vi "eec 6700 Perform Test in Manual Mode.vi"() -> ()   [LabVIEW 2014]
doc: "Configures the instrument in Manual mode and starts the test. The test meter data output is read from the instrument.\nPress stop button to end the test.\n\nNote : \n1.In firmware version 1.06, Enable Surge-Drop Mode is a system parameter (common for all steps and memory. Change in mode affect all steps and memory)\n\n2. In the firmware version 2.0 and above ,Enable Surge-Drop Mode can be used only in the Program Mode. And it can be used as a step parameter."
uses:
  <instrlib>/eec 6700/eec 6700.lvlib
panel:
  in  "Timeout (10000 ms)":u32=10000
  in  "Stop":bool
  in  "Frequency High Limit (500 Hz)":dbl=500.0 min=0.0 max=500.0 format="%.1f"
  in  "Frequency Low Limit (40 Hz)":dbl=40.0 min=0.0 max=500.0 format="%.1f"
  in  "End Angle: (0)":i32 min=0 max=359
  in  "Start Angle (0)":i32 min=0 max=359
  in  "Voltage Low Limit (0 V)":dbl min=0.0 max=400.0 format="%.1f"
  in  "Voltage High Limit (300 V)":dbl=300.0 min=0.0 max=400.0 format="%.1f"
  out "Test Meter Data Output":T1 {"Frequency (Hz)" format="%.1f"; "Voltage (V)" format="%.1f"; "RMS Current (A)" format="%.3f"; "Power (W)" format="%.1f"; "Peak Current (A)" format="%.1f"; "Power Factor" format="%.3f"; "Timer (s)" format="%.1f"}
  out "Status Byte Register Cluster":T2
  in  "Enable Surge Drop (F:Disable)":bool
  in  "Memory (1)":i32=1 min=1 max=50 step=1
  in  "Output AC Voltage Frequency (60  Hz)":dbl=60.0 min=45.0 max=500.0 format="%.1p"
  in  "Current High Limit (0 A)":dbl min=0.0 max=36.8 format="%.3f"
  in  "Output AC Voltage (115 V)":dbl=115.0 min=0.0 max=300.0 format="%.1f"
  in  "Voltage Range Mode (1:Auto)":u16(ring)=1 items=["High", "Auto"]
  in  "Surge Drop Duration (0 ms)":dbl min=0.0 max=99.0
  in  "Surge Drop Start Time (0 ms)":dbl min=0.0 max=99.0
  in  "Surge Drop Voltage (100 V)":dbl=100.0 min=0.0 max=300.0 format="%.1f"
  in  "Enable  Continuous Surge-Drop (F:Disable)":bool
  in  "Enable Over Current Fold Back (F:Disable)":bool
  in  "VISA resource name":refnum<visa-resource-name>="COM1"
  out "Error Out":errorcluster
  # "eec 6700 Manual MODE - EXAMPLE"
  # "Note :\n1. Configure the Parameters (Select the instrument VISA resource, voltage etc.,)\n2. Run this VI"
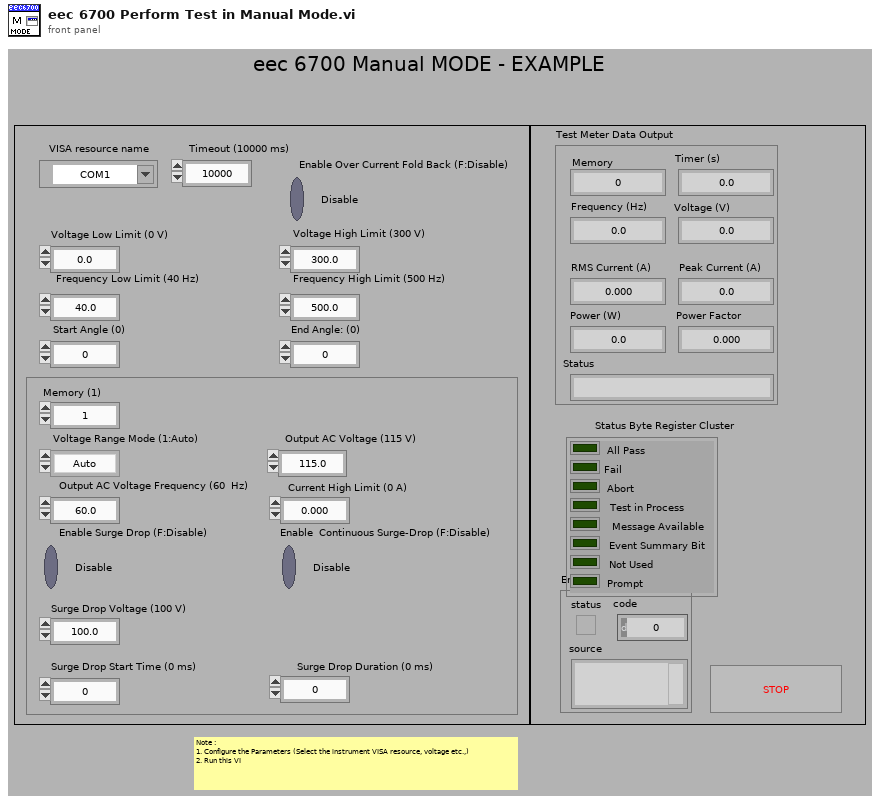
[diagram p1: front panel]
types:
  T1 = cluster{"Memory":dbl, "Timer (s)":dbl, "Frequency (Hz)":dbl, "Voltage (V)":dbl, "RMS Current (A)":dbl, "Peak Current (A)":dbl, "Power (W)":dbl, "Power Factor":dbl, "Status":string}
  T2 = cluster{"All Pass":bool, "Fail":bool, "Abort":bool, "Test in Process":bool, "Message Available":bool, "Event Summary Bit":bool, "Not Used":bool, "Prompt":bool}
  T3 = cluster{"Baud Rate":u32, "Parity":u16, "Data Bits":u16, "Stop Bits":u16, "Flow Control":u16}
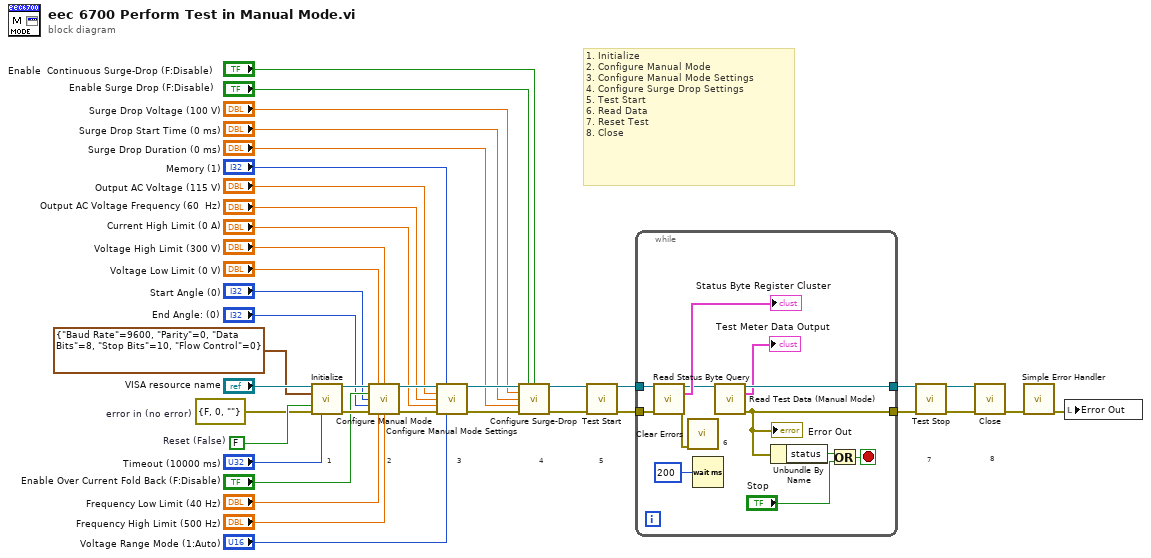
[diagram p0: block diagram]
diagram:
  w35 = errorcluster {"status"=FALSE, "code"=0, "source"=""}  # error in (no error)
  w36 = FALSE  # Reset (False)
  # "7"
  # "5"
  # "4"
  # "8"
  # "1. Initialize\n2. Configure Manual Mode\n3. Configure Manual Mode Settings\n4. Configure Surge Drop Settings\n5. Test Start\n6. Read Data\n7. Reset Test\n8. Close"
  # "3"
  # "2"
  # "1"
  n1 = call <instrlib>:"Initialize.vi"("VISA resource name"="VISA resource name", "Serial Configuration"=T3 {"Baud Rate"=9600, "Parity"=0, "Data Bits"=8, "Stop Bits"=10, "Flow Control"=0}, "Reset (True)"=w36, "error in (no error)"=w35, "Timeout (10000 ms)"="Timeout (10000 ms)") -> ("VISA resource name out"=w31:refnum<visa-resource-name>, "error out"=w33:errorcluster)  [unwired: 9 in]
  n2 = call <instrlib>:"Configure Manual Mode.vi"("VISA resource name"=w31, "Voltage Low Limit (0 V)"="Voltage Low Limit (0 V)", "Voltage High Limit (300 V)"="Voltage High Limit (300 V)", "Enable Over Current Fold Back (F:Disable)"="Enable Over Current Fold Back (F:Disable)", "Start Angle (0)"="Start Angle (0)", "End Angle: (0)"="End Angle: (0)", "error in (no error)"=w33, "Frequency Low Limit (40 Hz)"="Frequency Low Limit (40 Hz)", "Frequency High Limit (500 Hz)"="Frequency High Limit (500 Hz)") -> ("VISA resource name out"=w32:refnum<visa-resource-name>, "error out"=w34:errorcluster)  [unwired: 5 in]
  n3 = call <instrlib>:"Configure Manual Mode Settings.vi"("VISA resource name"=w32, "Memory (1)"="Memory (1)", "Output AC Voltage (115 V)"="Output AC Voltage (115 V)", "Output AC Voltage Frequency (60  Hz)"="Output AC Voltage Frequency (60  Hz)", "Current High Limit (0 A)"="Current High Limit (0 A)", "error in (no error)"=w34, "Voltage Range Mode (1:Auto)"="Voltage Range Mode (1:Auto)") -> ("VISA resource name out"=w29:refnum<visa-resource-name>, "error out"=w30:errorcluster)  [unwired: 7 in]
  n4 = call <instrlib>:"Configure Surge-Drop.vi"("VISA resource name"=w29, "Enable Surge Drop (F:Disable)"="Enable Surge Drop (F:Disable)", "Enable  Continuous Surge Drop (F:Disable)"="Enable  Continuous Surge-Drop (F:Disable)", "Surge Drop Voltage (100 V)"="Surge Drop Voltage (100 V)", "Surge Drop Start Time (0 ms)"="Surge Drop Start Time (0 ms)", "Surge Drop Duration (0 ms)"="Surge Drop Duration (0 ms)", "error in (no error)"=w30) -> ("VISA resource name out"=w5:refnum<visa-resource-name>, "error out"=w6:errorcluster)  [unwired: 7 in]
  n5 = call <instrlib>:"Test Start.vi"("VISA resource name"=w5, "error in (no error)"=w6) -> ("VISA resource name out"=w20:refnum<visa-resource-name>, "error out"=w19:errorcluster)  [unwired: 12 in]
  n6 = while {
    tunnel: w20 -> [w50]
    tunnel: w19 -> [w49]
    tunnel: [w46] -> w18
    tunnel: [w40] -> w15
    stop <- w41 stop-if-true
    # "6"
    n7 = call <instrlib>:"Read Status Byte Query.vi"("VISA resource name"=w50, "error in (no error)"=w49) -> ("VISA resource name out"=w47:refnum<visa-resource-name>, "Status Byte Register"=→"Status Byte Register Cluster":T2, "error out"=w39:errorcluster)  [unwired: 11 in]
    n8 = call <vilib>:"Clear Errors.vi"("error in (no error)"=w39) -> ()  [unwired: 5 in, 2 out]
    n9 = Wait (ms)(milliseconds to wait=u32 200) -> ()  [unwired: 1 out]
    n10 = call <instrlib>:"Read Test Data (Manual Mode).vi"("VISA resource name"=w47) -> ("VISA resource name out"=w46:refnum<visa-resource-name>, "Test Meter Data Output"=→"Test Meter Data Output":T1, "error out"=w40:errorcluster)  [unwired: 12 in]
    "Error Out" <- w40
    n11 = Unbundle By Name(w40) -> ("status"=w43:bool)
    n12 = Or(x=w43, y="Stop") -> (x .or. y?=w41:bool)
  }
  n13 = call <instrlib>:"Test Stop.vi"("VISA resource name"=w18, "error in (no error)"=w15) -> ("VISA resource name out"=w17:refnum<visa-resource-name>, "error out"=w16:errorcluster)  [unwired: 12 in]
  n14 = call <instrlib>:"Close.vi"("VISA resource name"=w17, "error in (no error)"=w16) -> ("error out"=w38:errorcluster)  [unwired: 13 in]
  n15 = call <vilib>:"Simple Error Handler.vi"("error in (no error)"=w38) -> ("error out"=w2:errorcluster)  [unwired: 4 in, 4 out]
  n16 = local write "Error Out"(w2) -> ()
